vi "Query Slit Speed.vi"(0 "VISA resource name":refnum<visa-resource-name>, 1 "Slit (Front/Axial Entrance)":T1, 3 "error in (no error)":errorcluster, 4 "Mono System # (0)":T2) -> (7 "VISA resource name out":refnum<visa-resource-name>, 9 "Frequency":dbl[unit], 10 "error out":errorcluster)   [LabVIEW 2009, in "JY-SPEX-TRIAX.lvlib"]
doc: "Queries the rate at which the slits will move."
uses:
  JY-SPEX-TRIAX.lvlib
  controls.llb/Monochromator System Number.ctl
  controls.llb/Slits.ctl
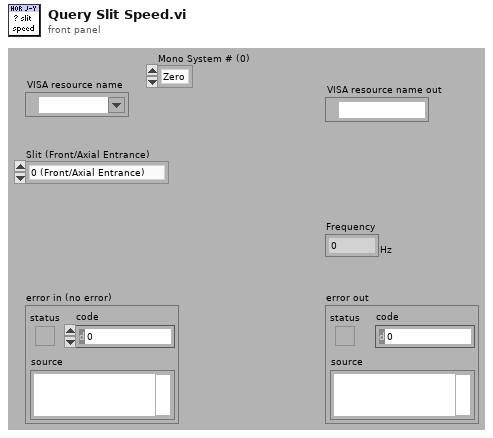
[diagram p1: front panel]
types:
  T1 = typedef "JY-SPEX-TRIAX.lvlib/Slits.ctl" = enum16{"0 (Front/Axial Entrance)", "1 (Side/Lateral Entrance)", "2 (Front/Axial Exit)", "3 (Side/Lateral Exit)"}
  T2 = typedef "JY-SPEX-TRIAX.lvlib/Monochromator System Number.ctl" = enum16{"Zero", "One"}
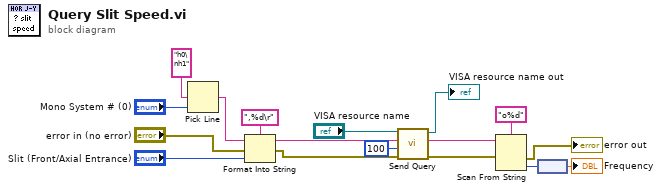
[diagram p0: block diagram]
diagram:
  n1 = Pick Line(multi-line string="h0\nh1", line index="Mono System # (0)") -> (output string=w15:string)  [unwired: 1 out]
  n2 = Format Into String(format string=",%d\r", initial string=w15, error in="error in (no error)", "Slit (Front/Axial Entrance)") -> (resulting string=w13:string, error out=w10:errorcluster)
  n3 = call "Send Query.vi"("error in (no error)"=w10, "byte count"=u32 100, "write buffer"=w13, "VISA resource name"="VISA resource name") -> ("error out"=w4:errorcluster, "read buffer"=w7:string, "VISA resource name out"=→"VISA resource name out":refnum<visa-resource-name>)  [unwired: 5 out]
  n4 = Scan From String(format string="o%d", input string=w7, error in=w4) -> (error out=→"error out":errorcluster, output 1=w3:i32)  [unwired: 1 in, 3 out]
  n5 = node(w3) -> (→"Frequency":dbl[unit])
